vi "Write Bypass_.vi"(8 "error in (no error)":errorcluster, 10 "Bypass?":bool, 11 "Change Denuded Bypass State in":refnum<class "Change Denuded Bypass State.lvclass">) -> (0 "error out":errorcluster, 3 "Change Denuded Bypass State out":refnum<class "Change Denuded Bypass State.lvclass">)   [LabVIEW 2014, in "Change Denuded Bypass State.lvclass"]
uses:
  Change Denuded Bypass State.lvclass
  Change Denuded Bypass State.lvclass/Change Denuded Bypass State.ctl
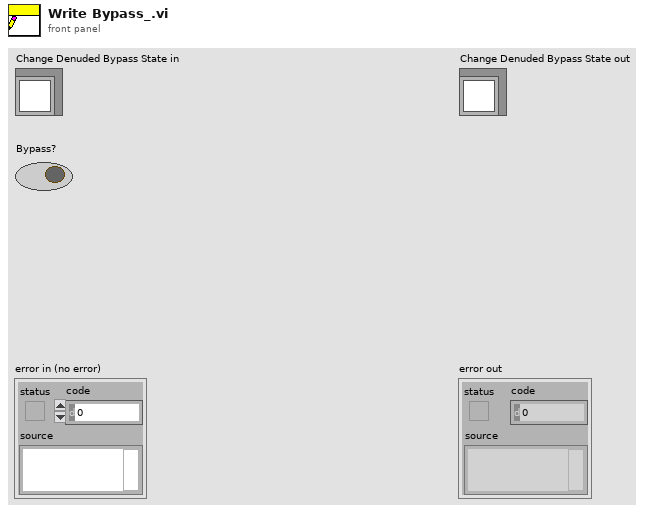
[diagram p1: front panel]
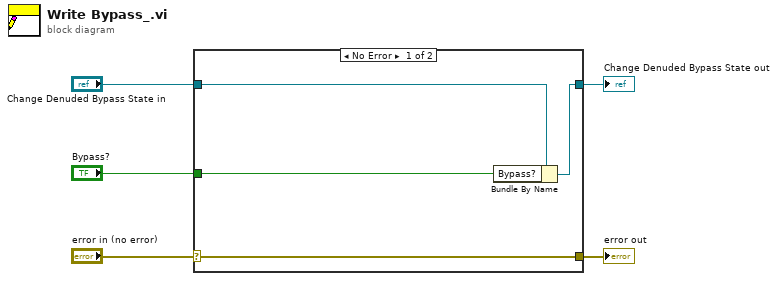
[diagram p0: block diagram]
diagram:
  n1 = case shown="No Error" "error in (no error)" {
    selector: "error in (no error)" -> [w9 w10]
    tunnel: [w9 w10] -> w4
    tunnel: [w7 w11] -> w2
    tunnel: "Change Denuded Bypass State in" -> [w8 w11]
    tunnel: "Bypass?" -> [w6 _]
    frame No Error {
      n2 = Bundle By Name(cluster=w8, "Bypass?"=w6) -> (w7:refnum<class "Change Denuded Bypass State.lvclass">)
    }
    frame Error {
    }
  }
  "error out" <- w4
  "Change Denuded Bypass State out" <- w2
